vi "Initialize Washing Queue.vi"(3 "error in (no error)":errorcluster) -> (7 "queue out":refnum<queue>, 10 "error out":errorcluster)   [LabVIEW 2015]
uses:
  Washing Control Cluster.ctl
  States of Washing.ctl
panel:
  in  "Washing Control Cluster":T1
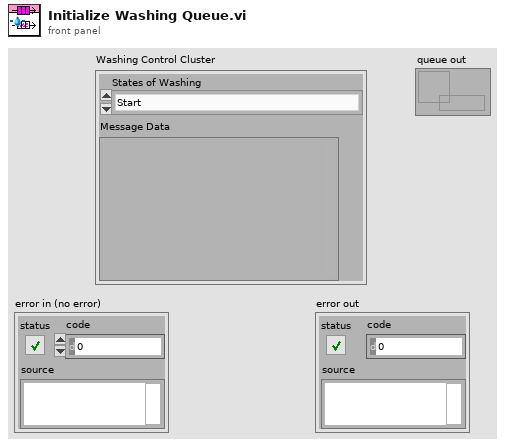
[diagram p1: front panel]
types:
  T1 = typedef "Washing Control Cluster.ctl" = cluster{"Message Data":variant, "States of Washing":T2}
  T2 = typedef "States of Washing.ctl" = enum16{"Start", "Under Body Wash", "Bug Remover", "Pre-Soak", "High Pressure Wax", "Low Pressure Wax", "Spot Free Rinse", "Tire Shine Foam", "Air Dry", "End", "Initialize"}
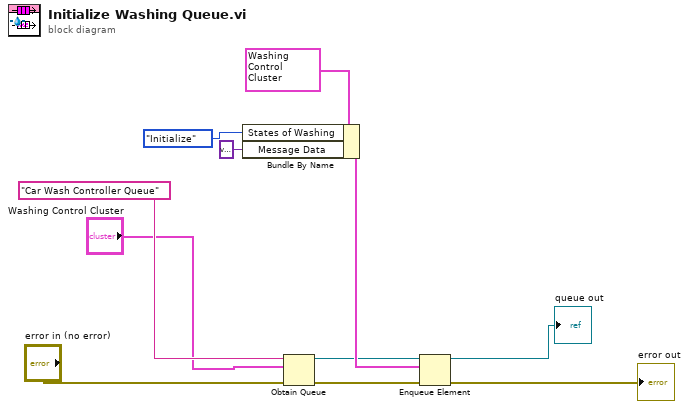
[diagram p0: block diagram]
diagram:
  n1 = Bundle By Name(cluster=T1 {"Message Data"=variant, "States of Washing"=enum."Initialize"} ("Washing Control Cluster"), "States of Washing"=States_of_Washing."Initialize", "Message Data"=variant) -> (w8:T1)
  n2 = Obtain Queue(name (unnamed)="Car Wash Controller Queue", element data type="Washing Control Cluster", error in (no error)="error in (no error)") -> (queue out=w7:refnum<queue>, error out=w2:errorcluster)  [unwired: 2 in, 1 out]
  n3 = Enqueue Element(queue=w7, element=w8, error in (no error)=w2) -> (queue out=→"queue out":refnum<queue>, error out=→"error out":errorcluster)  [unwired: 1 in, 1 out]
